vi "Teardown.vi"(11 "Dev Actor in":refnum<class "Dev Actor.lvclass">) -> (3 "Dev Actor out":refnum<class "Dev Actor.lvclass">)   [LabVIEW 2021, in "Dev Actor.lvlib" / "Dev Actor.lvclass"]
uses:
  Dev Actor.lvclass
  Dev Actor.lvclass/Dev Actor.ctl
  Queue Actor/Queue Actor.lvclass
  Dev Panel/Dev Panel.lvclass
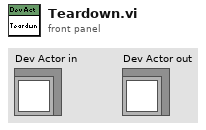
[diagram p1: front panel]
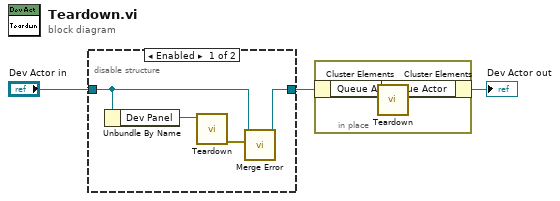
[diagram p0: block diagram]
diagram:
  n1 = disable-structure shown="Enabled" {
    disable-tunnel: "Dev Actor in" -> [w5 w8]
    disable-tunnel: [w4 w8] -> w1
    frame Enabled {
      n2 = Unbundle By Name(w5) -> ("Dev Panel"=w7:refnum<class "Dev Panel.lvclass">)
      n3 = call "Teardown.vi"("Dev Actor Panel in"=w7) -> ("error out"=w6:errorcluster)  [unwired: 10 in]
      n4 = call-dynamic "Merge Error.vi"("Error"=w6, "Dev Actor in"=w5) -> ("Dev Actor out"=w4:refnum<class "Dev Actor.lvclass">)  [unwired: 9 in]
    }
    frame Disabled {
    }
  }
  n5 = in-place {
    n6 = in-place-cluster #1(w1) -> ("Queue Actor"=w10:refnum<class "Queue Actor.lvclass">)
    n7 = call-dynamic "Teardown.vi"("Teardown in"=w10) -> ("Teardown out"=w9:refnum<class "Queue Actor.lvclass">)  [unwired: 10 in]
    n8 = in-place-cluster #1("Queue Actor"=w9) -> (→"Dev Actor out":refnum<class "Dev Actor.lvclass">)
  }
